vi "MT Get Axis Software P Now.vi"(10 "pValue":i32, 11 "AObj":u16) -> (2 "pValue out":i32, 3 "function return":i32)   [LabVIEW 2014, in "MT_API.lvlib"]
doc: "MT_API INT32 __stdcall MT_Get_Axis_Software_P_Now(WORD AObj,INT32* pValue);"
uses:
  MT_API.lvlib
  MT_API.dll
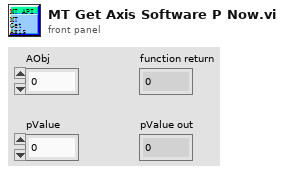
[diagram p1: front panel]
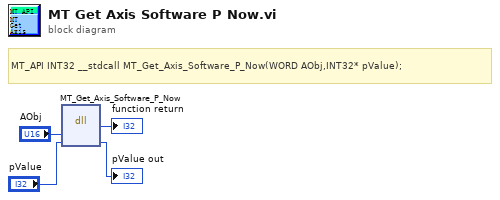
[diagram p0: block diagram]
diagram:
  # "MT_API INT32 __stdcall MT_Get_Axis_Software_P_Now(WORD AObj,INT32* pValue);"
  n1 = dll-call lib="E:/Projects/LabView/MT_API/MT_API.*" fn="MT_Get_Axis_Software_P_Now"("AObj"="AObj", "pValue"="pValue") -> (→"function return":i32, "pValue"=→"pValue out":i32)  [unwired: 4 in, 2 out]
